vi "cycling_inflation.vi"() -> ()   [LabVIEW 2014]
doc: "This VI demonstrates the individual configuration of settings in I/W, W/I, and continuous operation modes.\n\nThis VI is not meant to be used with infusion-only models. \n\nNotes:\n(1) If continuous mode is selected, infuse volumes/rates will be used."
uses:
  <instrlib>/KD Scientific 2XX Series/KD Scientific 2XX Series.lvlib
panel:
  in  "Number of Cycles":i32
  in  "number of steps":i32
  out "Units":string
  out "Delivered Volume":dbl
  in  "stop":bool
  out "Status":T1
  in  "Baud Rate (9600)":u32(ring)=9600 items=["300"=300, "1200"=1200, "2400"=2400, "4800"=4800, "9600"=9600]
  in  "Withdrawal Settings":T2={"Flow Rate (5)"=5.0, "Volume (10)"=10.0, "Volume Units (ml)"=enum."milliliters (ml)", "Rate Units (ml/min.)"=enum."milliliters per minute (ml/min.)"} {"Volume (10)" format="%#.3g"}
  in  "Diameter (8.75 mm)":dbl=8.75
  in  "Infusion Settings":T2={"Flow Rate (5)"=5.0, "Volume (10)"=10.0, "Volume Units (ml)"=enum."milliliters (ml)", "Rate Units (ml/min.)"=enum."milliliters per minute (ml/min.)"}
  in  "Address (0)":i32 format="%0.0f"
  in  "error in (no error)":errorcluster
  in  "VISA resource name":refnum<visa-resource-name>="COM1"
  # "RS-232 Settings"
  # "General Settings"
  # "Pump Status"
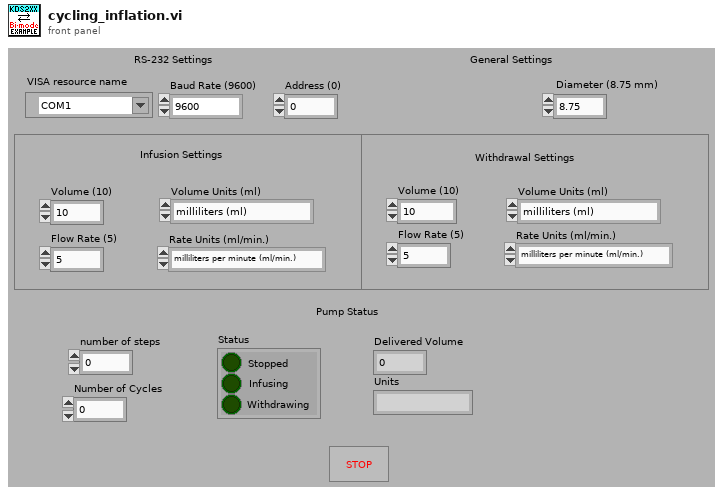
[diagram p1: front panel]
types:
  T1 = cluster{"Stopped":bool, "Infusing":bool, "Withdrawing":bool}
  T2 = cluster{"Flow Rate (5)":dbl, "Volume (10)":dbl, "Volume Units (ml)":enum16{"milliliters (ml)", "microliters (ul)"}, "Rate Units (ml/min.)":enum16{"milliliters per minute (ml/min.)", "milliliters per hour (ml/hr.)", "microliters per minute (ul/min.)", "microliters per hour (ul/hr.)"}}
  T3 = enum16{"milliliters per minute (ml/min.)", "milliliters per hour (ml/hr.)", "microliters per minute (ul/min.)", "microliters per hour (ul/hr.)"}
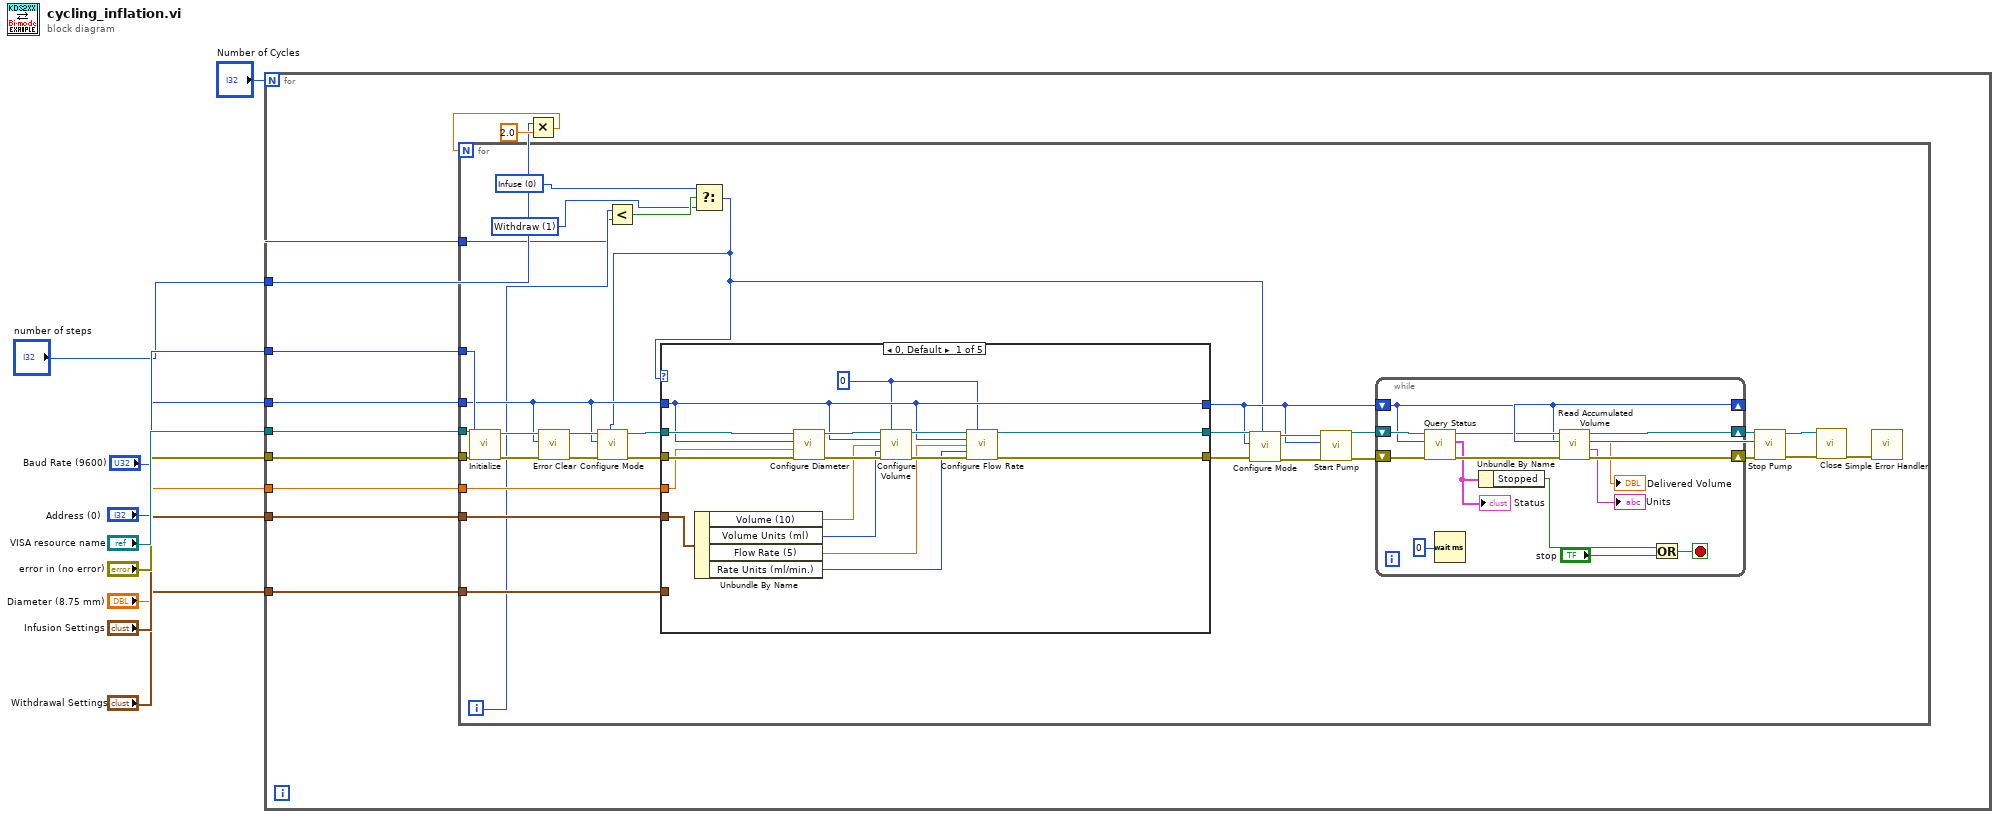
[diagram p0: block diagram]
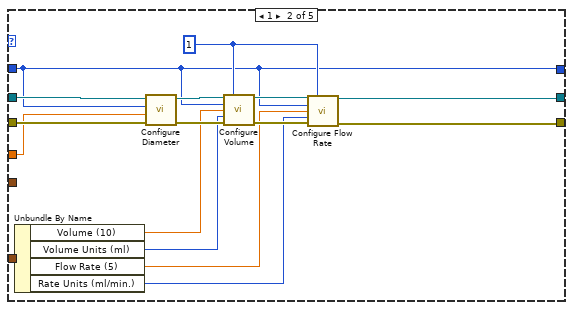
[diagram p2: hidden frame]
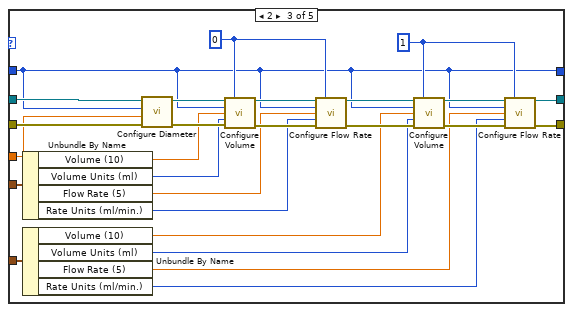
[diagram p3: hidden frame]
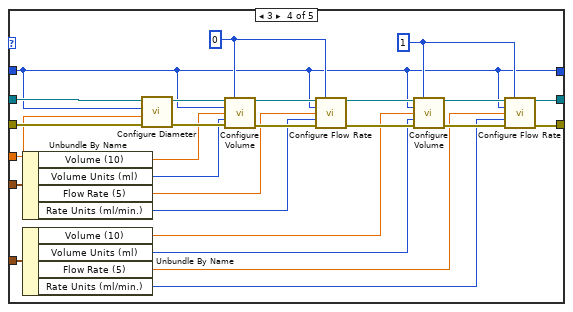
[diagram p4: hidden frame]
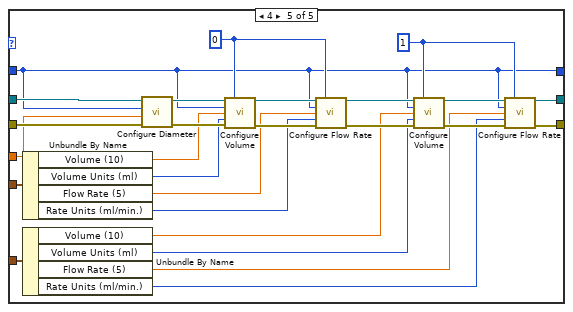
[diagram p5: hidden frame]
diagram:
  n1 = for {
    N: "Number of Cycles" -> [_]
    tunnel: "VISA resource name" -> [w19]
    tunnel: "error in (no error)" -> [w18]
    tunnel: "Infusion Settings" -> [w17]
    tunnel: "Withdrawal Settings" -> [w16]
    tunnel: "Diameter (8.75 mm)" -> [w15]
    tunnel: "Baud Rate (9600)" -> [w14]
    tunnel: "Address (0)" -> [w13]
    tunnel: "number of steps" -> [w10]
    n2 = Multiply(x=w10, y=2.0) -> (x*y=w11:dbl)
    n3 = for {
      N: w11 -> [_]
      tunnel: w19 -> [w51]
      tunnel: w18 -> [w50]
      tunnel: w17 -> [w45]
      tunnel: w16 -> [w44]
      tunnel: w15 -> [w43]
      tunnel: w14 -> [w38]
      tunnel: w13 -> [w26]
      tunnel: w10 -> [w24]
      i -> [w25]
      w21 = u16 1 items=["Withdraw"=1]
      w22 = u16 0 items=["Infuse"] ("Mode (infuse)")
      n4 = call <instrlib>:"Initialize.vi"("error in (no error)"=w50, "Baud Rate (9600)"=w38, "VISA resource name"=w51) -> ("error out"=w28:errorcluster, "VISA resource name out"=w27:refnum<visa-resource-name>)  [unwired: 7 in]
      n5 = call <instrlib>:"Error Clear.vi"("error in (no error)"=w28, "Address (0)"=w26, "VISA resource name"=w27) -> ("error out"=w29:errorcluster, "VISA resource name out"=w30:refnum<visa-resource-name>)  [unwired: 6 in, 1 out]
      n6 = Less?(x=w25, y=w24) -> (x < y?=w23:bool)
      n7 = Select(t=w22, s=w23, f=w21) -> (s? t:f=w20:u16)
      n8 = call <instrlib>:"Configure Mode.vi"("Mode (infuse)"=w20, "error in (no error)"=w29, "Address (0)"=w26, "VISA resource name"=w30) -> ("error out"=w32:errorcluster, "VISA resource name out"=w31:refnum<visa-resource-name>)  [unwired: 6 in]
      n9 = case shown="0, Default" w20 {
        tunnel: w45 -> [w61 _ w109 w135 w161]
        tunnel: w44 -> [_ w83 w108 w134 w160]
        tunnel: w31 -> [w67 w82 w107 w133 w159]
        tunnel: w32 -> [w66 w78 w106 w132 w158]
        tunnel: w43 -> [w60 w74 w89 w115 w141]
        tunnel: [w59 w68 w84 w110 w136] -> w33
        tunnel: w26 -> [w59 w68 w84 w110 w136]
        tunnel: [w54 w79 w86 w112 w138] -> w37
        tunnel: [w53 w75 w85 w111 w137] -> w36
        frame 0, Default {
          w52 = 0
          n10 = Unbundle By Name(w61) -> ("Volume (10)"=w58:dbl, "Volume Units (ml)"=w57:enum16{"milliliters (ml)", "microliters (ul)"}, "Flow Rate (5)"=w56:dbl, "Rate Units (ml/min.)"=w55:T3)
          n11 = call <instrlib>:"Configure Diameter.vi"("error in (no error)"=w66, "Diameter (8.75 mm)"=w60, "Address (0)"=w59, "VISA resource name"=w67) -> ("error out"=w64:errorcluster, "VISA resource name out"=w65:refnum<visa-resource-name>)  [unwired: 6 in]
          n12 = call <instrlib>:"Configure Volume.vi"("VISA resource name"=w65, "Mode (infuse)"=w52, "Address (0)"=w59, "Volume (100)"=w58, "Units (0: milliliters)"=w57, "error in (no error)"=w64) -> ("VISA resource name out"=w63:refnum<visa-resource-name>, "error out"=w62:errorcluster)  [unwired: 8 in]
          n13 = call <instrlib>:"Configure Flow Rate.vi"("VISA resource name"=w63, "Mode (infuse)"=w52, "Address (0)"=w59, "Flow Rate (5)"=w56, "Units (0: milliliters per minute)"=w55, "error in (no error)"=w62) -> ("VISA resource name out"=w54:refnum<visa-resource-name>, "error out"=w53:errorcluster)  [unwired: 8 in]
        }
        frame 1 {
          w69 = 1
          n14 = Unbundle By Name(w83) -> ("Volume (10)"=w73:dbl, "Volume Units (ml)"=w72:enum16{"milliliters (ml)", "microliters (ul)"}, "Flow Rate (5)"=w71:dbl, "Rate Units (ml/min.)"=w70:T3)
          n15 = call <instrlib>:"Configure Diameter.vi"("error in (no error)"=w78, "Diameter (8.75 mm)"=w74, "Address (0)"=w68, "VISA resource name"=w82) -> ("error out"=w77:errorcluster, "VISA resource name out"=w81:refnum<visa-resource-name>)  [unwired: 6 in]
          n16 = call <instrlib>:"Configure Volume.vi"("VISA resource name"=w81, "Mode (infuse)"=w69, "Address (0)"=w68, "Volume (100)"=w73, "Units (0: milliliters)"=w72, "error in (no error)"=w77) -> ("VISA resource name out"=w80:refnum<visa-resource-name>, "error out"=w76:errorcluster)  [unwired: 8 in]
          n17 = call <instrlib>:"Configure Flow Rate.vi"("VISA resource name"=w80, "Mode (infuse)"=w69, "Address (0)"=w68, "Flow Rate (5)"=w71, "Units (0: milliliters per minute)"=w70, "error in (no error)"=w76) -> ("VISA resource name out"=w79:refnum<visa-resource-name>, "error out"=w75:errorcluster)  [unwired: 8 in]
        }
        frame 2 {
          w87 = 1
          w88 = 0
          n18 = Unbundle By Name(w109) -> ("Volume (10)"=w97:dbl, "Volume Units (ml)"=w96:enum16{"milliliters (ml)", "microliters (ul)"}, "Flow Rate (5)"=w95:dbl, "Rate Units (ml/min.)"=w94:T3)
          n19 = Unbundle By Name(w108) -> ("Volume (10)"=w93:dbl, "Volume Units (ml)"=w92:enum16{"milliliters (ml)", "microliters (ul)"}, "Flow Rate (5)"=w91:dbl, "Rate Units (ml/min.)"=w90:T3)
          n20 = call <instrlib>:"Configure Diameter.vi"("error in (no error)"=w106, "Diameter (8.75 mm)"=w89, "Address (0)"=w84, "VISA resource name"=w107) -> ("error out"=w101:errorcluster, "VISA resource name out"=w105:refnum<visa-resource-name>)  [unwired: 6 in]
          n21 = call <instrlib>:"Configure Volume.vi"("VISA resource name"=w105, "Mode (infuse)"=w88, "Address (0)"=w84, "Volume (100)"=w97, "Units (0: milliliters)"=w96, "error in (no error)"=w101) -> ("VISA resource name out"=w104:refnum<visa-resource-name>, "error out"=w100:errorcluster)  [unwired: 8 in]
          n22 = call <instrlib>:"Configure Flow Rate.vi"("VISA resource name"=w104, "Mode (infuse)"=w88, "Address (0)"=w84, "Flow Rate (5)"=w95, "Units (0: milliliters per minute)"=w94, "error in (no error)"=w100) -> ("VISA resource name out"=w103:refnum<visa-resource-name>, "error out"=w99:errorcluster)  [unwired: 8 in]
          n23 = call <instrlib>:"Configure Volume.vi"("VISA resource name"=w103, "Mode (infuse)"=w87, "Address (0)"=w84, "Volume (100)"=w93, "Units (0: milliliters)"=w92, "error in (no error)"=w99) -> ("VISA resource name out"=w102:refnum<visa-resource-name>, "error out"=w98:errorcluster)  [unwired: 8 in]
          n24 = call <instrlib>:"Configure Flow Rate.vi"("VISA resource name"=w102, "Mode (infuse)"=w87, "Address (0)"=w84, "Flow Rate (5)"=w91, "Units (0: milliliters per minute)"=w90, "error in (no error)"=w98) -> ("VISA resource name out"=w86:refnum<visa-resource-name>, "error out"=w85:errorcluster)  [unwired: 8 in]
        }
        frame 3 {
          w113 = 1
          w114 = 0
          n25 = Unbundle By Name(w135) -> ("Volume (10)"=w123:dbl, "Volume Units (ml)"=w122:enum16{"milliliters (ml)", "microliters (ul)"}, "Flow Rate (5)"=w121:dbl, "Rate Units (ml/min.)"=w120:T3)
          n26 = Unbundle By Name(w134) -> ("Volume (10)"=w119:dbl, "Volume Units (ml)"=w118:enum16{"milliliters (ml)", "microliters (ul)"}, "Flow Rate (5)"=w117:dbl, "Rate Units (ml/min.)"=w116:T3)
          n27 = call <instrlib>:"Configure Diameter.vi"("error in (no error)"=w132, "Diameter (8.75 mm)"=w115, "Address (0)"=w110, "VISA resource name"=w133) -> ("error out"=w127:errorcluster, "VISA resource name out"=w131:refnum<visa-resource-name>)  [unwired: 6 in]
          n28 = call <instrlib>:"Configure Volume.vi"("VISA resource name"=w131, "Mode (infuse)"=w114, "Address (0)"=w110, "Volume (100)"=w123, "Units (0: milliliters)"=w122, "error in (no error)"=w127) -> ("VISA resource name out"=w130:refnum<visa-resource-name>, "error out"=w126:errorcluster)  [unwired: 8 in]
          n29 = call <instrlib>:"Configure Flow Rate.vi"("VISA resource name"=w130, "Mode (infuse)"=w114, "Address (0)"=w110, "Flow Rate (5)"=w121, "Units (0: milliliters per minute)"=w120, "error in (no error)"=w126) -> ("VISA resource name out"=w129:refnum<visa-resource-name>, "error out"=w125:errorcluster)  [unwired: 8 in]
          n30 = call <instrlib>:"Configure Volume.vi"("VISA resource name"=w129, "Mode (infuse)"=w113, "Address (0)"=w110, "Volume (100)"=w119, "Units (0: milliliters)"=w118, "error in (no error)"=w125) -> ("VISA resource name out"=w128:refnum<visa-resource-name>, "error out"=w124:errorcluster)  [unwired: 8 in]
          n31 = call <instrlib>:"Configure Flow Rate.vi"("VISA resource name"=w128, "Mode (infuse)"=w113, "Address (0)"=w110, "Flow Rate (5)"=w117, "Units (0: milliliters per minute)"=w116, "error in (no error)"=w124) -> ("VISA resource name out"=w112:refnum<visa-resource-name>, "error out"=w111:errorcluster)  [unwired: 8 in]
        }
        frame 4 {
          w139 = 1
          w140 = 0
          n32 = Unbundle By Name(w161) -> ("Volume (10)"=w149:dbl, "Volume Units (ml)"=w148:enum16{"milliliters (ml)", "microliters (ul)"}, "Flow Rate (5)"=w147:dbl, "Rate Units (ml/min.)"=w146:T3)
          n33 = Unbundle By Name(w160) -> ("Volume (10)"=w145:dbl, "Volume Units (ml)"=w144:enum16{"milliliters (ml)", "microliters (ul)"}, "Flow Rate (5)"=w143:dbl, "Rate Units (ml/min.)"=w142:T3)
          n34 = call <instrlib>:"Configure Diameter.vi"("error in (no error)"=w158, "Diameter (8.75 mm)"=w141, "Address (0)"=w136, "VISA resource name"=w159) -> ("error out"=w153:errorcluster, "VISA resource name out"=w157:refnum<visa-resource-name>)  [unwired: 6 in]
          n35 = call <instrlib>:"Configure Volume.vi"("VISA resource name"=w157, "Mode (infuse)"=w140, "Address (0)"=w136, "Volume (100)"=w149, "Units (0: milliliters)"=w148, "error in (no error)"=w153) -> ("VISA resource name out"=w156:refnum<visa-resource-name>, "error out"=w152:errorcluster)  [unwired: 8 in]
          n36 = call <instrlib>:"Configure Flow Rate.vi"("VISA resource name"=w156, "Mode (infuse)"=w140, "Address (0)"=w136, "Flow Rate (5)"=w147, "Units (0: milliliters per minute)"=w146, "error in (no error)"=w152) -> ("VISA resource name out"=w155:refnum<visa-resource-name>, "error out"=w151:errorcluster)  [unwired: 8 in]
          n37 = call <instrlib>:"Configure Volume.vi"("VISA resource name"=w155, "Mode (infuse)"=w139, "Address (0)"=w136, "Volume (100)"=w145, "Units (0: milliliters)"=w144, "error in (no error)"=w151) -> ("VISA resource name out"=w154:refnum<visa-resource-name>, "error out"=w150:errorcluster)  [unwired: 8 in]
          n38 = call <instrlib>:"Configure Flow Rate.vi"("VISA resource name"=w154, "Mode (infuse)"=w139, "Address (0)"=w136, "Flow Rate (5)"=w143, "Units (0: milliliters per minute)"=w142, "error in (no error)"=w150) -> ("VISA resource name out"=w138:refnum<visa-resource-name>, "error out"=w137:errorcluster)  [unwired: 8 in]
        }
      }
      n39 = call <instrlib>:"Configure Mode.vi"("Mode (infuse)"=w20, "error in (no error)"=w36, "Address (0)"=w33, "VISA resource name"=w37) -> ("error out"=w34:errorcluster, "VISA resource name out"=w35:refnum<visa-resource-name>)  [unwired: 6 in]
      n40 = call <instrlib>:"Start Pump.vi"("error in (no error)"=w34, "Address (0)"=w33, "VISA resource name"=w35) -> ("error out"=w48:errorcluster, "VISA resource name out"=w49:refnum<visa-resource-name>)  [unwired: 7 in]
      n41 = while {
        shift-right: [w164] -> w42
        shift-left: w33 -> [w164]
        shift-right: [w166] -> w47
        shift-left: w49 -> [w172]
        shift-right: [w165] -> w46
        shift-left: w48 -> [w173]
        stop <- w170 stop-if-true
        n42 = call <instrlib>:"Query Status.vi"("error in (no error)"=w173, "Address (0)"=w164, "VISA resource name"=w172) -> ("error out"=w175:errorcluster, "Status"=w171:T1, "VISA resource name out"=w167:refnum<visa-resource-name>)  [unwired: 6 in]
        "Status" <- w171
        n43 = Wait (ms)(milliseconds to wait=u32 0) -> ()  [unwired: 1 out]
        n44 = Unbundle By Name(w171) -> ("Stopped"=w169:bool)
        n45 = call <instrlib>:"Read Accumulated Volume.vi"("error in (no error)"=w175, "Address (0)"=w164, "VISA resource name"=w167) -> ("error out"=w165:errorcluster, "Units"=→"Units":string, "Delivered Volume"=→"Delivered Volume":dbl, "VISA resource name out"=w166:refnum<visa-resource-name>)  [unwired: 5 in]
        n46 = Or(x=w169, y="stop") -> (x .or. y?=w170:bool)
      }
      n47 = call <instrlib>:"Stop Pump.vi"("error in (no error)"=w46, "Address (0)"=w42, "VISA resource name"=w47) -> ("error out"=w40:errorcluster, "VISA resource name out"=w39:refnum<visa-resource-name>)  [unwired: 7 in]
      n48 = call <instrlib>:"Close.vi"("error in (no error)"=w40, "VISA resource name"=w39) -> ("error out"=w41:errorcluster)  [unwired: 9 in]
      n49 = call <vilib>:"Simple Error Handler.vi"("error in (no error)"=w41) -> ()  [unwired: 4 in, 5 out]
    }
  }
